vi "GetVariable.vi"(1 "Vaste käsk":string="E", 2 "VISA resource name":refnum<visa-resource-name>) -> (0 "Väljund":string)   [LabVIEW 2012]
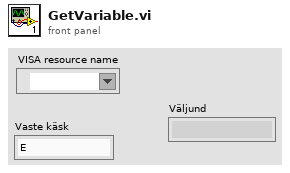
[diagram p1: front panel]
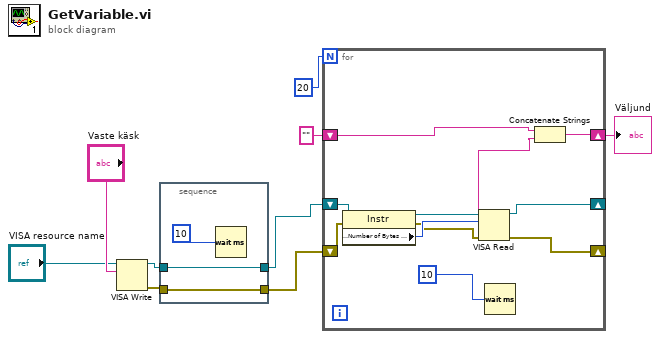
[diagram p0: block diagram]
diagram:
  n1 = VISA Write(VISA resource name="VISA resource name", write buffer="Vaste käsk") -> (VISA resource name out=w8:refnum<visa-resource-name>, error out=w7:errorcluster)  [unwired: 1 in, 1 out]
  n2 = stacked-sequence {
    tunnel: w7 -> [w12]
    tunnel: [w12] -> w6
    tunnel: w8 -> [w11]
    tunnel: [w11] -> w5
    frame #0 {
      n3 = Wait (ms)(milliseconds to wait=u32 10 ("delay Input")) -> ()  [unwired: 1 out]
    }
  }
  n4 = for {
    N: 20 -> [_]
    shift-right: [w13] -> w2
    shift-left: "" -> [w14]
    shift-right: [w18] -> _
    shift-left: w5 -> [w16]
    shift-right: [w17] -> _
    shift-left: w6 -> [w19]
    n5 = property class="Instr"(reference=w16, error in=w19) -> (reference out=w23:refnum<visa-resource-name>, error out=w21:errorcluster, "Serial Settings:Number of Bytes at Serial Port"=w22:u32)
    n6 = VISA Read(VISA resource name=w23, byte count=w22, error in (no error)=w21) -> (VISA resource name out=w18:refnum<visa-resource-name>, read buffer=w15:string, error out=w17:errorcluster)  [unwired: 1 out]
    n7 = Wait (ms)(milliseconds to wait=u32 10 ("delay Input 2")) -> ()  [unwired: 1 out]
    n8 = Concatenate Strings(w14, w15) -> (w13:string)
  }
  "Väljund" <- w2
